vi "Decode OK_NG.vi"(11 "Boolean":bool) -> (1 "result":string, 2 "OK":bool, 3 "NG":bool caption="OK")   [LabVIEW 2016]
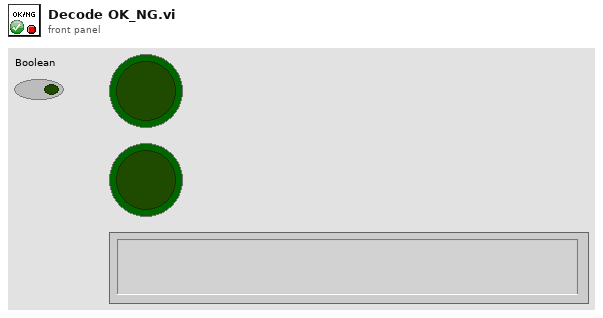
[diagram p1: front panel]
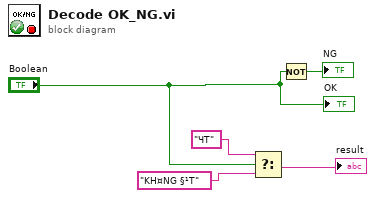
[diagram p0: block diagram]
diagram:
  n1 = Select(t="ЧT", s="Boolean", f="KH¤NG §¹T") -> (s? t:f=→"result":string)
  n2 = Not(x="Boolean") -> (.not. x?=→"NG":bool)
  "OK" <- "Boolean"
